vi "Angles.vi"(1 "Y2":dbl format="%#_13g", 2 "X2":dbl format="%#_13g", 3 "Y1":dbl format="%#_13g", 4 "X1":dbl format="%#_13g") -> (0 "Numeric":dbl=0.1234 format="%#_13g")   [LabVIEW 2016]
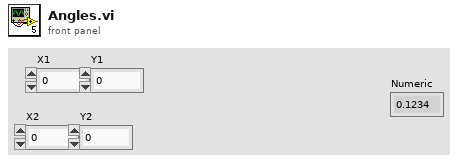
[diagram p1: front panel]
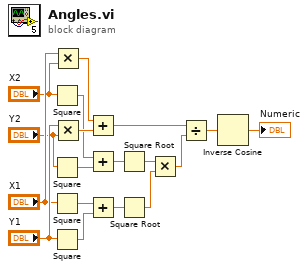
[diagram p0: block diagram]
diagram:
  n1 = Square(x="X2") -> (x^2=w15:dbl)
  n2 = Square(x="Y2") -> (x^2=w14:dbl)
  n3 = Square(x="X1") -> (x^2=w12:dbl)
  n4 = Square(x="Y1") -> (x^2=w11:dbl)
  n5 = Multiply(x="X1", y="X2") -> (x*y=w18:dbl)
  n6 = Multiply(x="Y1", y="Y2") -> (x*y=w17:dbl)
  n7 = Add(x=w18, y=w17) -> (x+y=w6:dbl)
  n8 = Add(x=w15, y=w14) -> (x+y=w16:dbl)
  n9 = Add(x=w12, y=w11) -> (x+y=w13:dbl)
  n10 = Square Root(x=w16) -> (sqrt(x)=w9:dbl)
  n11 = Square Root(x=w13) -> (sqrt(x)=w8:dbl)
  n12 = Multiply(x=w9, y=w8) -> (x*y=w7:dbl)
  n13 = Divide(x=w6, y=w7) -> (x/y=w5:dbl)
  n14 = Inverse Cosine(1:w5) -> (0:→"Numeric":dbl)
